vi "BSTNumericLimitTest.vi"() -> (0 "error out":errorcluster, 1 "Report Text":string, 2 "Numeric Measurement":dbl=25.89 format="%.2f")   [LabVIEW 2010]
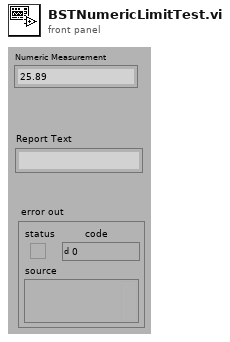
[diagram p1: front panel]
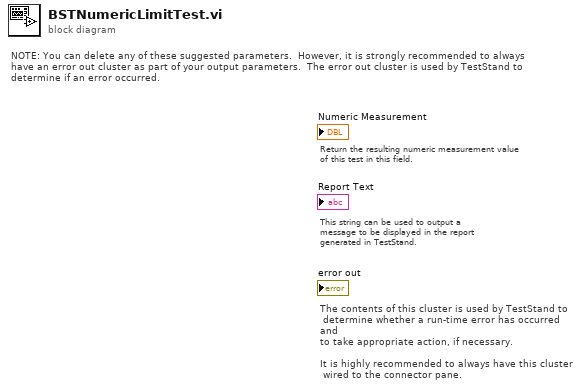
[diagram p0: block diagram]
diagram:
  # "Return the resulting numeric measurement value \nof this test in this field."
  # "The contents of this cluster is used by TestStand to\n determine whether a run-time error has occurred and\nto take appropriate action, if necessary.\n\nIt is highly recommended to always have this cluster\n wired to the connector pane."
  # "This string can be used to output a\nmessage to be displayed in the report\ngenerated in TestStand."
  # "NOTE: You can delete any of these suggested parameters.  However, it is strongly recommended to always have an error out cluster as part of your output parameters.  The error out cluster is used by TestStand to determine if an error occurred."
